vi "DownSampleData_MaxMin.vi"(8 "error in (no error)":errorcluster, 10 "Desired Sampling Rate":dbl=2000.0, 11 "Oversampled Values":waveform(sgl)[](array[waveform])) -> (0 "error out":errorcluster, 3 "Downsampled Data":waveform(sgl)[](array[waveform]))   [LabVIEW 2020]
doc: "This VI takes oversampled data and averages the data to downsample to the desired sampling rate. For instance, if data is captured at 2000 Hz for 1 second and the desired sampling rate is 50 Hz, every new data point is the result of averaging 40 data points (from the 2000 Hz data stream)."
panel:
  out "size(s)":i32
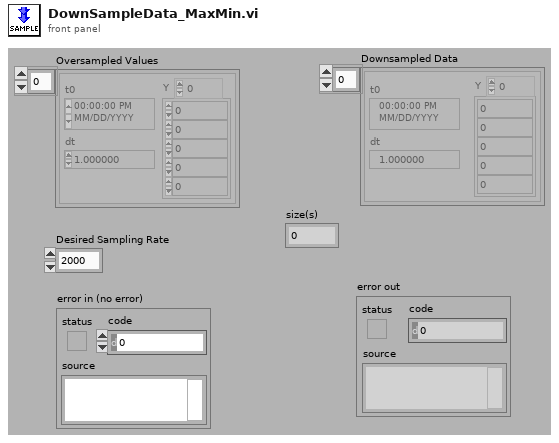
[diagram p1: front panel]
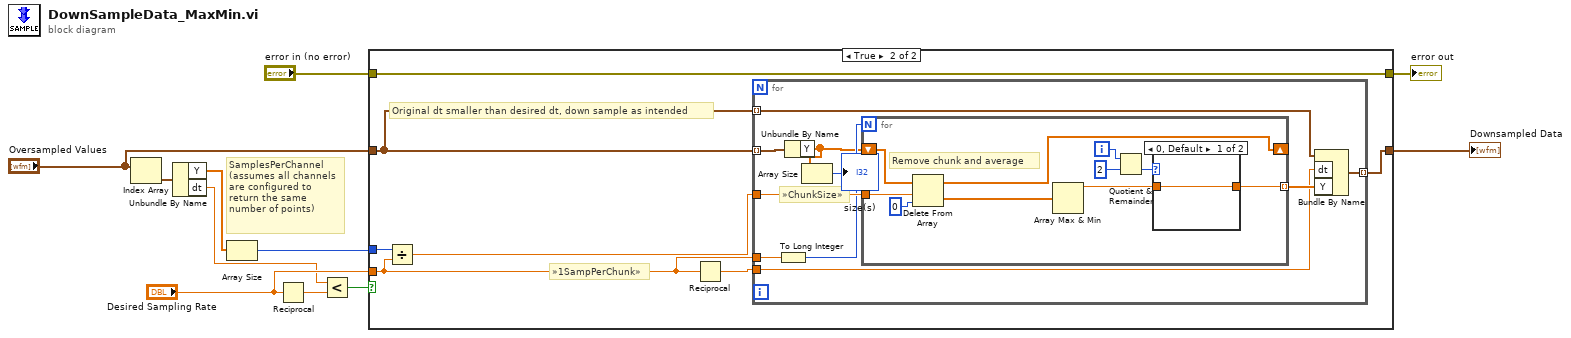
[diagram p0: block diagram]
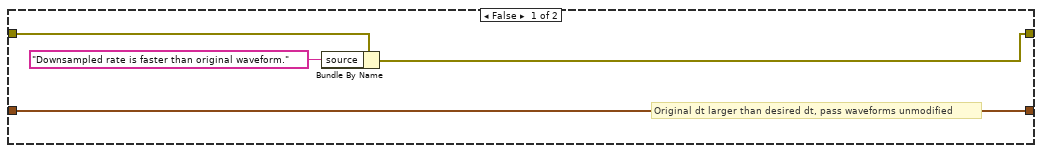
[diagram p2: hidden frame]
diagram:
  # "SamplesPerChannel\n(assumes all channels\nare configured to \nreturn the same \nnumber of points)"
  n1 = Index Array(array="Oversampled Values") -> (element=w9:waveform(sgl))  [unwired: 1 in]
  n2 = Unbundle By Name(w9) -> ("Y"=w8:sgl[], "dt"=w2:dbl)
  n3 = Array Size(array=w8) -> (size(s)=w7:i32)
  n4 = Reciprocal(x="Desired Sampling Rate") -> (1/x=w3:dbl)
  n5 = Less?(x=w2, y=w3) -> (x < y?=w1:bool)
  n6 = case shown="True" w1 {
    tunnel: "Desired Sampling Rate" -> [_ w21]
    tunnel: [w15 w19] -> w11
    tunnel: "Oversampled Values" -> [w15 w18]
    tunnel: w7 -> [_ w17]
    tunnel: [w13 w16] -> w6
    tunnel: "error in (no error)" -> [w14 w16]
    frame False {
      # "Original dt larger than desired dt, pass waveforms unmodified"
      n7 = Bundle By Name(cluster=w14, "source"="Downsampled rate is faster than original waveform.") -> (w13:errorcluster)
    }
    frame True {
      # "Original dt smaller than desired dt, down sample as intended"
      # "»1SampPerChunk»"
      n8 = Divide(x=w17, y=w21) -> (x/y=w22:dbl)
      n9 = Reciprocal(x=w21) -> (1/x=w20:dbl)
      n10 = for {
        tunnel: w18 -> [w32] mode=indexing
        tunnel: [w27] -> w19 mode=indexing
        tunnel: w21 -> [w31]
        tunnel: w22 -> [w30]
        tunnel: w20 -> [w28]
        tunnel: w18 -> [w26] mode=indexing
        # "»ChunkSize»"
        n11 = To Long Integer(number=w31) -> (32bit integer=w25:i32)
        n12 = Unbundle By Name(w32) -> ("Y"=w24:sgl[])
        n13 = Array Size(array=w24) -> (size(s)=→"size(s)":i32)
        n14 = for {
          N: w25 -> [_]
          tunnel: [w34] -> w29 mode=indexing
          shift-right: [w40] -> _
          shift-left: w24 -> [w41]
          tunnel: w30 -> [w39]
          i -> [w38]
          # "Remove chunk and average"
          n15 = Delete From Array(array=w41, length=w39, index=0) -> (deleted portion=w35:sgl[], array with subset deleted=w40:sgl[])
          n16 = Array Max & Min(array=w35) -> (max value=w33:sgl)  [unwired: 3 out]
          n17 = Quotient & Remainder(x=w38, y=2) -> (floor(x/y)=w36:i32)  [unwired: 1 out]
          n18 = case shown="0, Default" w36 {
            tunnel: [w43 w44] -> w34
            tunnel: w33 -> [w43 w44]
            frame 0, Default {
            }
            frame 1 {
            }
          }
        }
        n19 = Bundle By Name(cluster=w26, "dt"=w28, "Y"=w29) -> (w27:waveform(sgl))
      }
    }
  }
  "Downsampled Data" <- w11
  "error out" <- w6
